vi "servo.vi"() -> ()   [LabVIEW 2023]
uses:
  <vilib>/Platform/TimedLoop/XDataNode/timing_clust.ctl
  <vilib>/Platform/TimedLoop/XDataNode/nitl_modes.ctl
  <vilib>/Platform/TimedLoop/XDataNode/wakeup.ctl
  <vilib>/Instr/_visa.llb/VISA Configure Serial Port (Instr).vi
  <vilib>/Utility/file.llb/Write Delimited Spreadsheet (DBL).vi
  <vilib>/Utility/file.llb/Write Delimited Spreadsheet (string).vi
  C:/Users/Ali/Desktop/ServoMotor/utilitytools39.dll
  utilitytools39.dll
  <vilib>/platform/TimedLoop/XDataNode/XDataNode.xnode
  <vilib>/Platform/TimedLoop/XDataNode/XDNodeRunTimeDep.lvlib
panel:
  out "Part":string
  out "ServoType":string
  in  "Speed Test":enum32{"A", "B"}(radio)
  out "final":string[][](array[string])
  out "k":dbl[](array[numeric])
  out "resultOfStep":dbl[](array[numeric])
  out "results":dbl[][](array[numeric])
  in  "Export And Save Data":bool
  in  "Title:":string
  out "Type":string[](array[string])
  out "stop var":bool
  out "Command":string
  out "SelectedType":bool
  out "SelectedPort":bool
  in  "Servo Motor PartNumber":string
  in  "Servo Motor type":string(combo)
  out "String 2":string
  in  "Select  Port":refnum<visa-resource-name>
  out "On/Off":bool
  in  "stop":bool
  in  "start":bool
  in  "Angle (degree)":i32(knob)=9 min=9 max=21 step=1 scale=9.0..21.0
  in  "Torque (N.m)":i32(slide) min=0 max=12 step=1 scale=0.0..12.0
  in  "Select":T1(radio)=enum."Torque Test"
  out "Angle":dbl(knob) scale=180.0..-180.0 scale format="%#_6f"
  out "Current (mA)":dbl(knob) scale=0.0..5500.0 scale format="%#_6f"
  out "Speed (degree/s)":dbl(knob) scale=0.0..600.0 scale format="%#_6f"
  out "Voltage  (volt)":dbl(knob) scale=0.0..25.0 scale format="%#_6f"
  out "Torque (N.M)":dbl(knob) scale=0.0..40.0 scale format="%#3.2f"
  # "Pishgaman Sanat Tissan  - Servo Motor Tester"
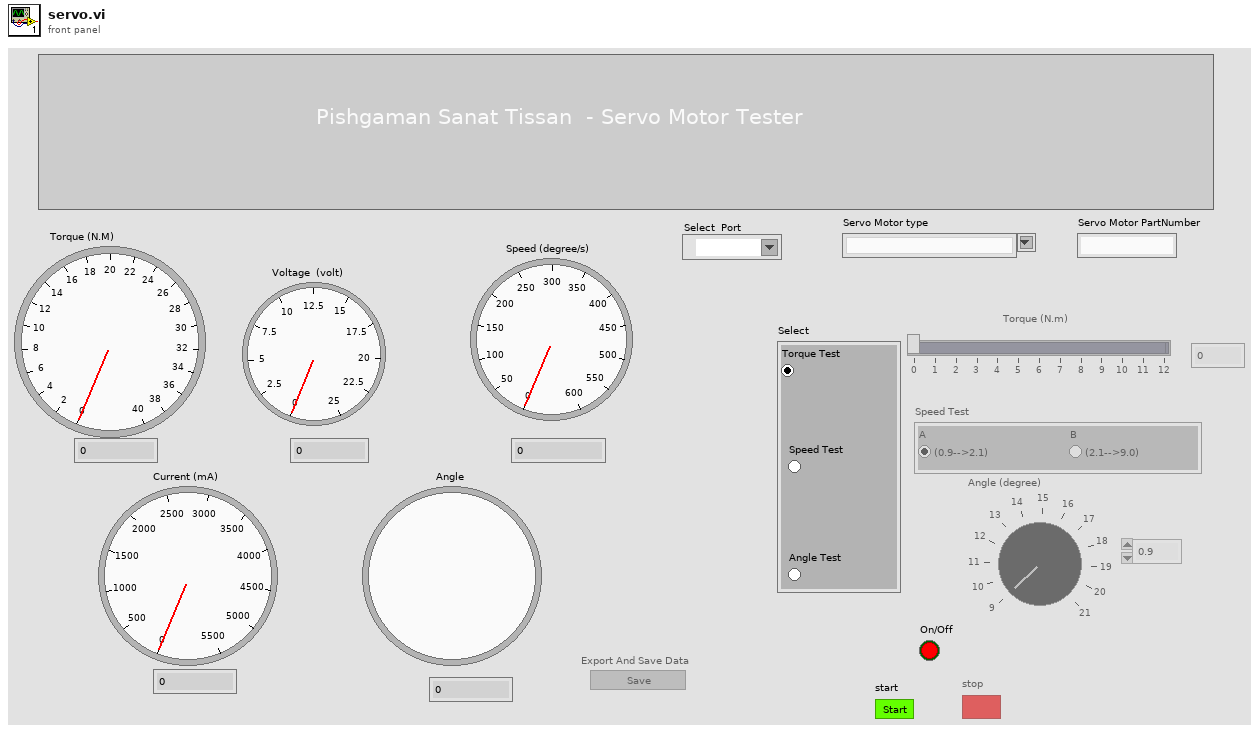
[diagram p1: front panel]
types:
  T1 = enum32{"No Selection", "Torque Test", "Speed Test", "Angle Test"}
  T2 = typedef "XDNodeRunTimeDep.lvlib/timing_clust.ctl" = cluster{"Expected End [f-1]":u64, "Actual End [f-1]":u64, "Finished Late? [f-1]":bool, "Expected End [i-1]":u64, "Actual End [i-1]":u64, "Finished Late? [i-1]":bool, "Expected Start [i]":u64, "Actual Start [i]":u64, "Expected Start [f]":u64, "Actual Start [f]":u64, "Source Name":string, "Structure Name":string, "Period":i64, "Deadline":i64, "Offset":i64, "Start":i64, "Priority":i32, "Timeout":i32, "Mode":T3, "Wakeup Reason":T4, "Error":errorcluster, "Source Type":string, "Secondary Source Type":string, "Global End Time":u64, "Global Start Time":u64, "Frame Duration":u64, "Iteration Duration":u64, "Assigned CPU":i32, "I/O Scan Engine Mode":u32}
  T3 = typedef "XDNodeRunTimeDep.lvlib/nitl_modes.ctl" = enum32{"No Change", "Process missed periods, maintain original phase", "Discard missed periods, maintain original phase", "Process missed periods, ignore original phase", "Discard missed periods, ignore original phase"}
  T4 = typedef "XDNodeRunTimeDep.lvlib/wakeup.ctl" = enum32{"Normal", "Aborted", "Asynchronous wakeup", "Timing source error", "Timed loop error", "Timeout"}
  T5 = typedef "LVDataSocketStatusTypeDef.ctl" = cluster{"Code":enum32{"Invalid Status", "Unconnected", "Active", "Idle", "Error", "Connecting"}, "Text":string}
  T6 = enum32{"Invalid Status", "Unconnected", "Active", "Idle", "Error", "Connecting"}
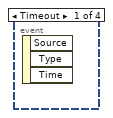
[diagram p2: hidden frame]
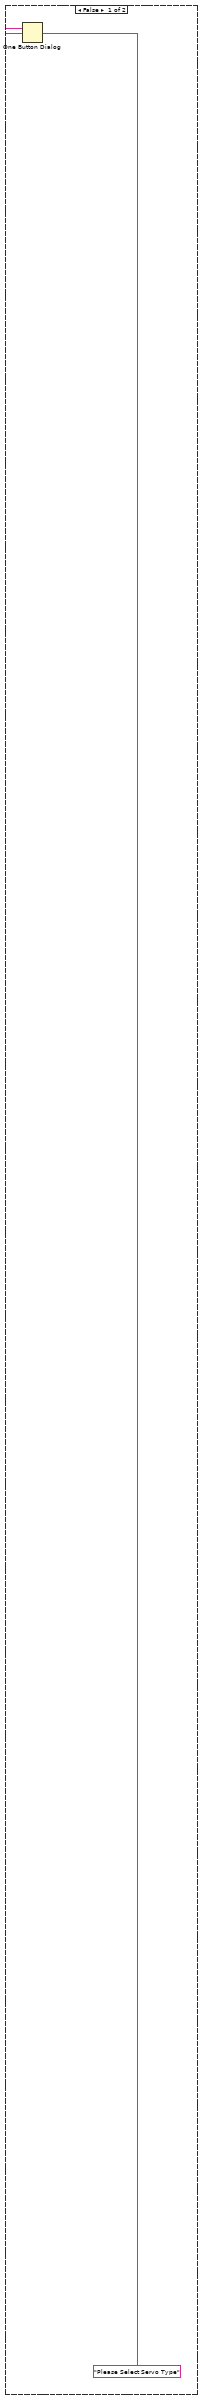
[diagram p4: hidden frame]
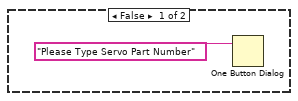
[diagram p5: hidden frame]
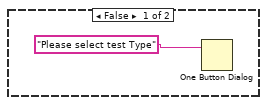
[diagram p6: hidden frame]
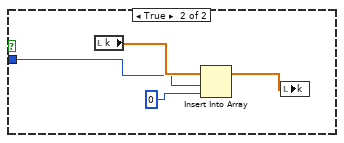
[diagram p7: hidden frame]
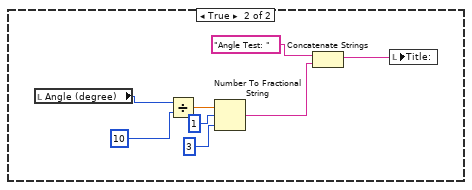
[diagram p12: hidden frame]
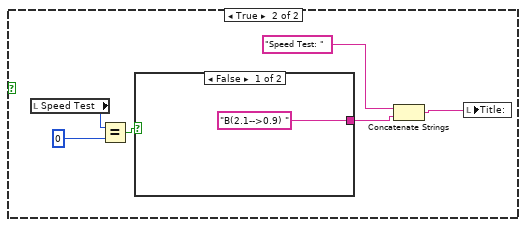
[diagram p13: hidden frame]
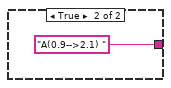
[diagram p14: hidden frame]
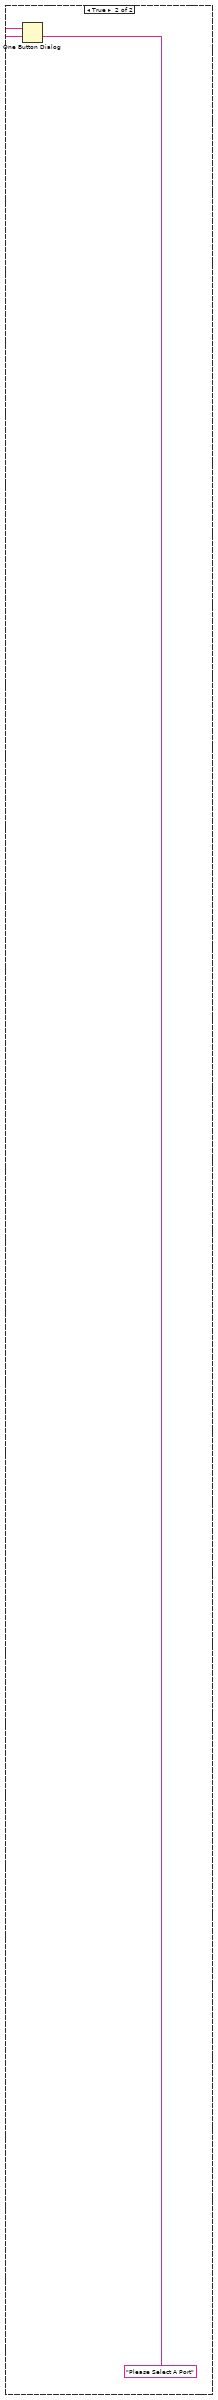
[diagram p17: hidden frame]
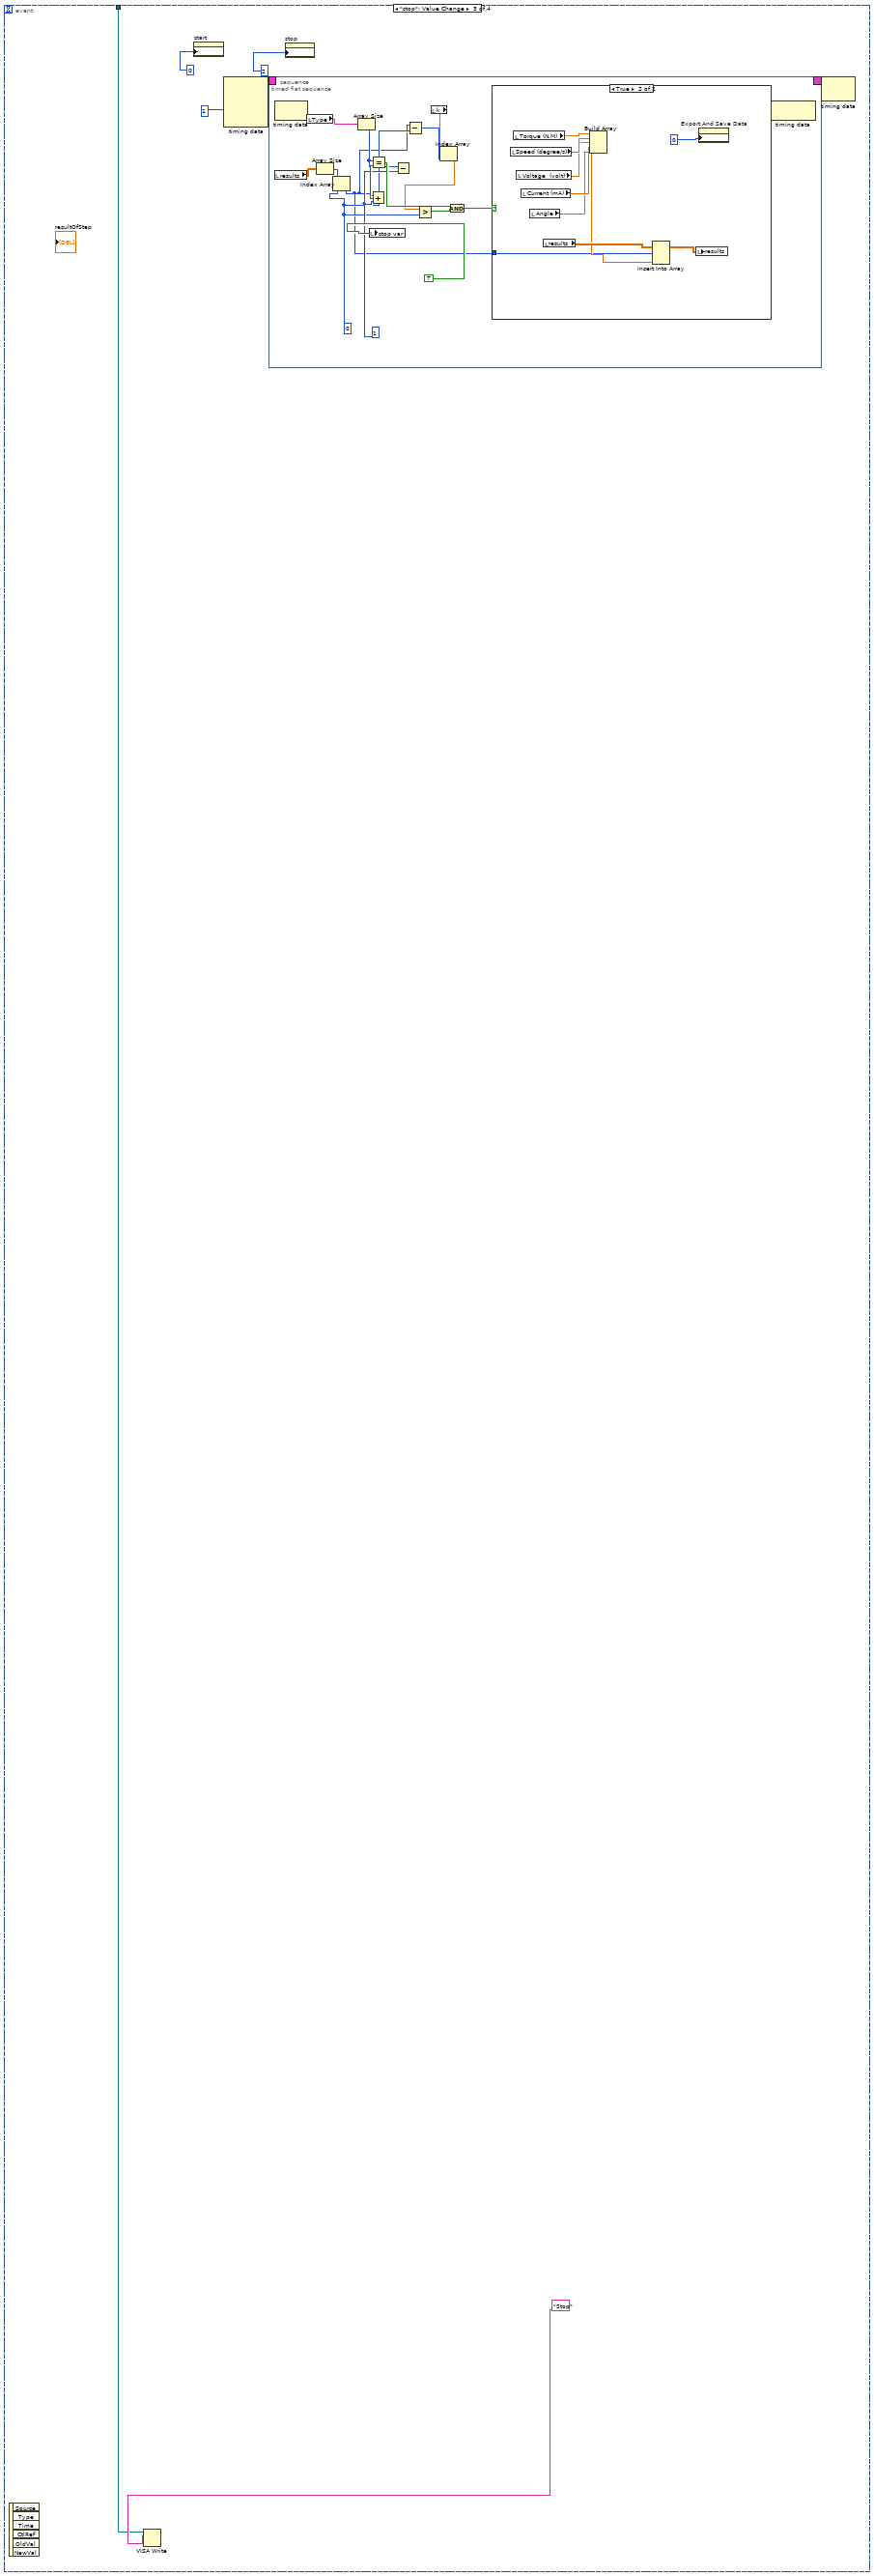
[diagram p18: hidden frame]
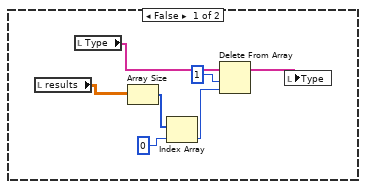
[diagram p19: hidden frame]
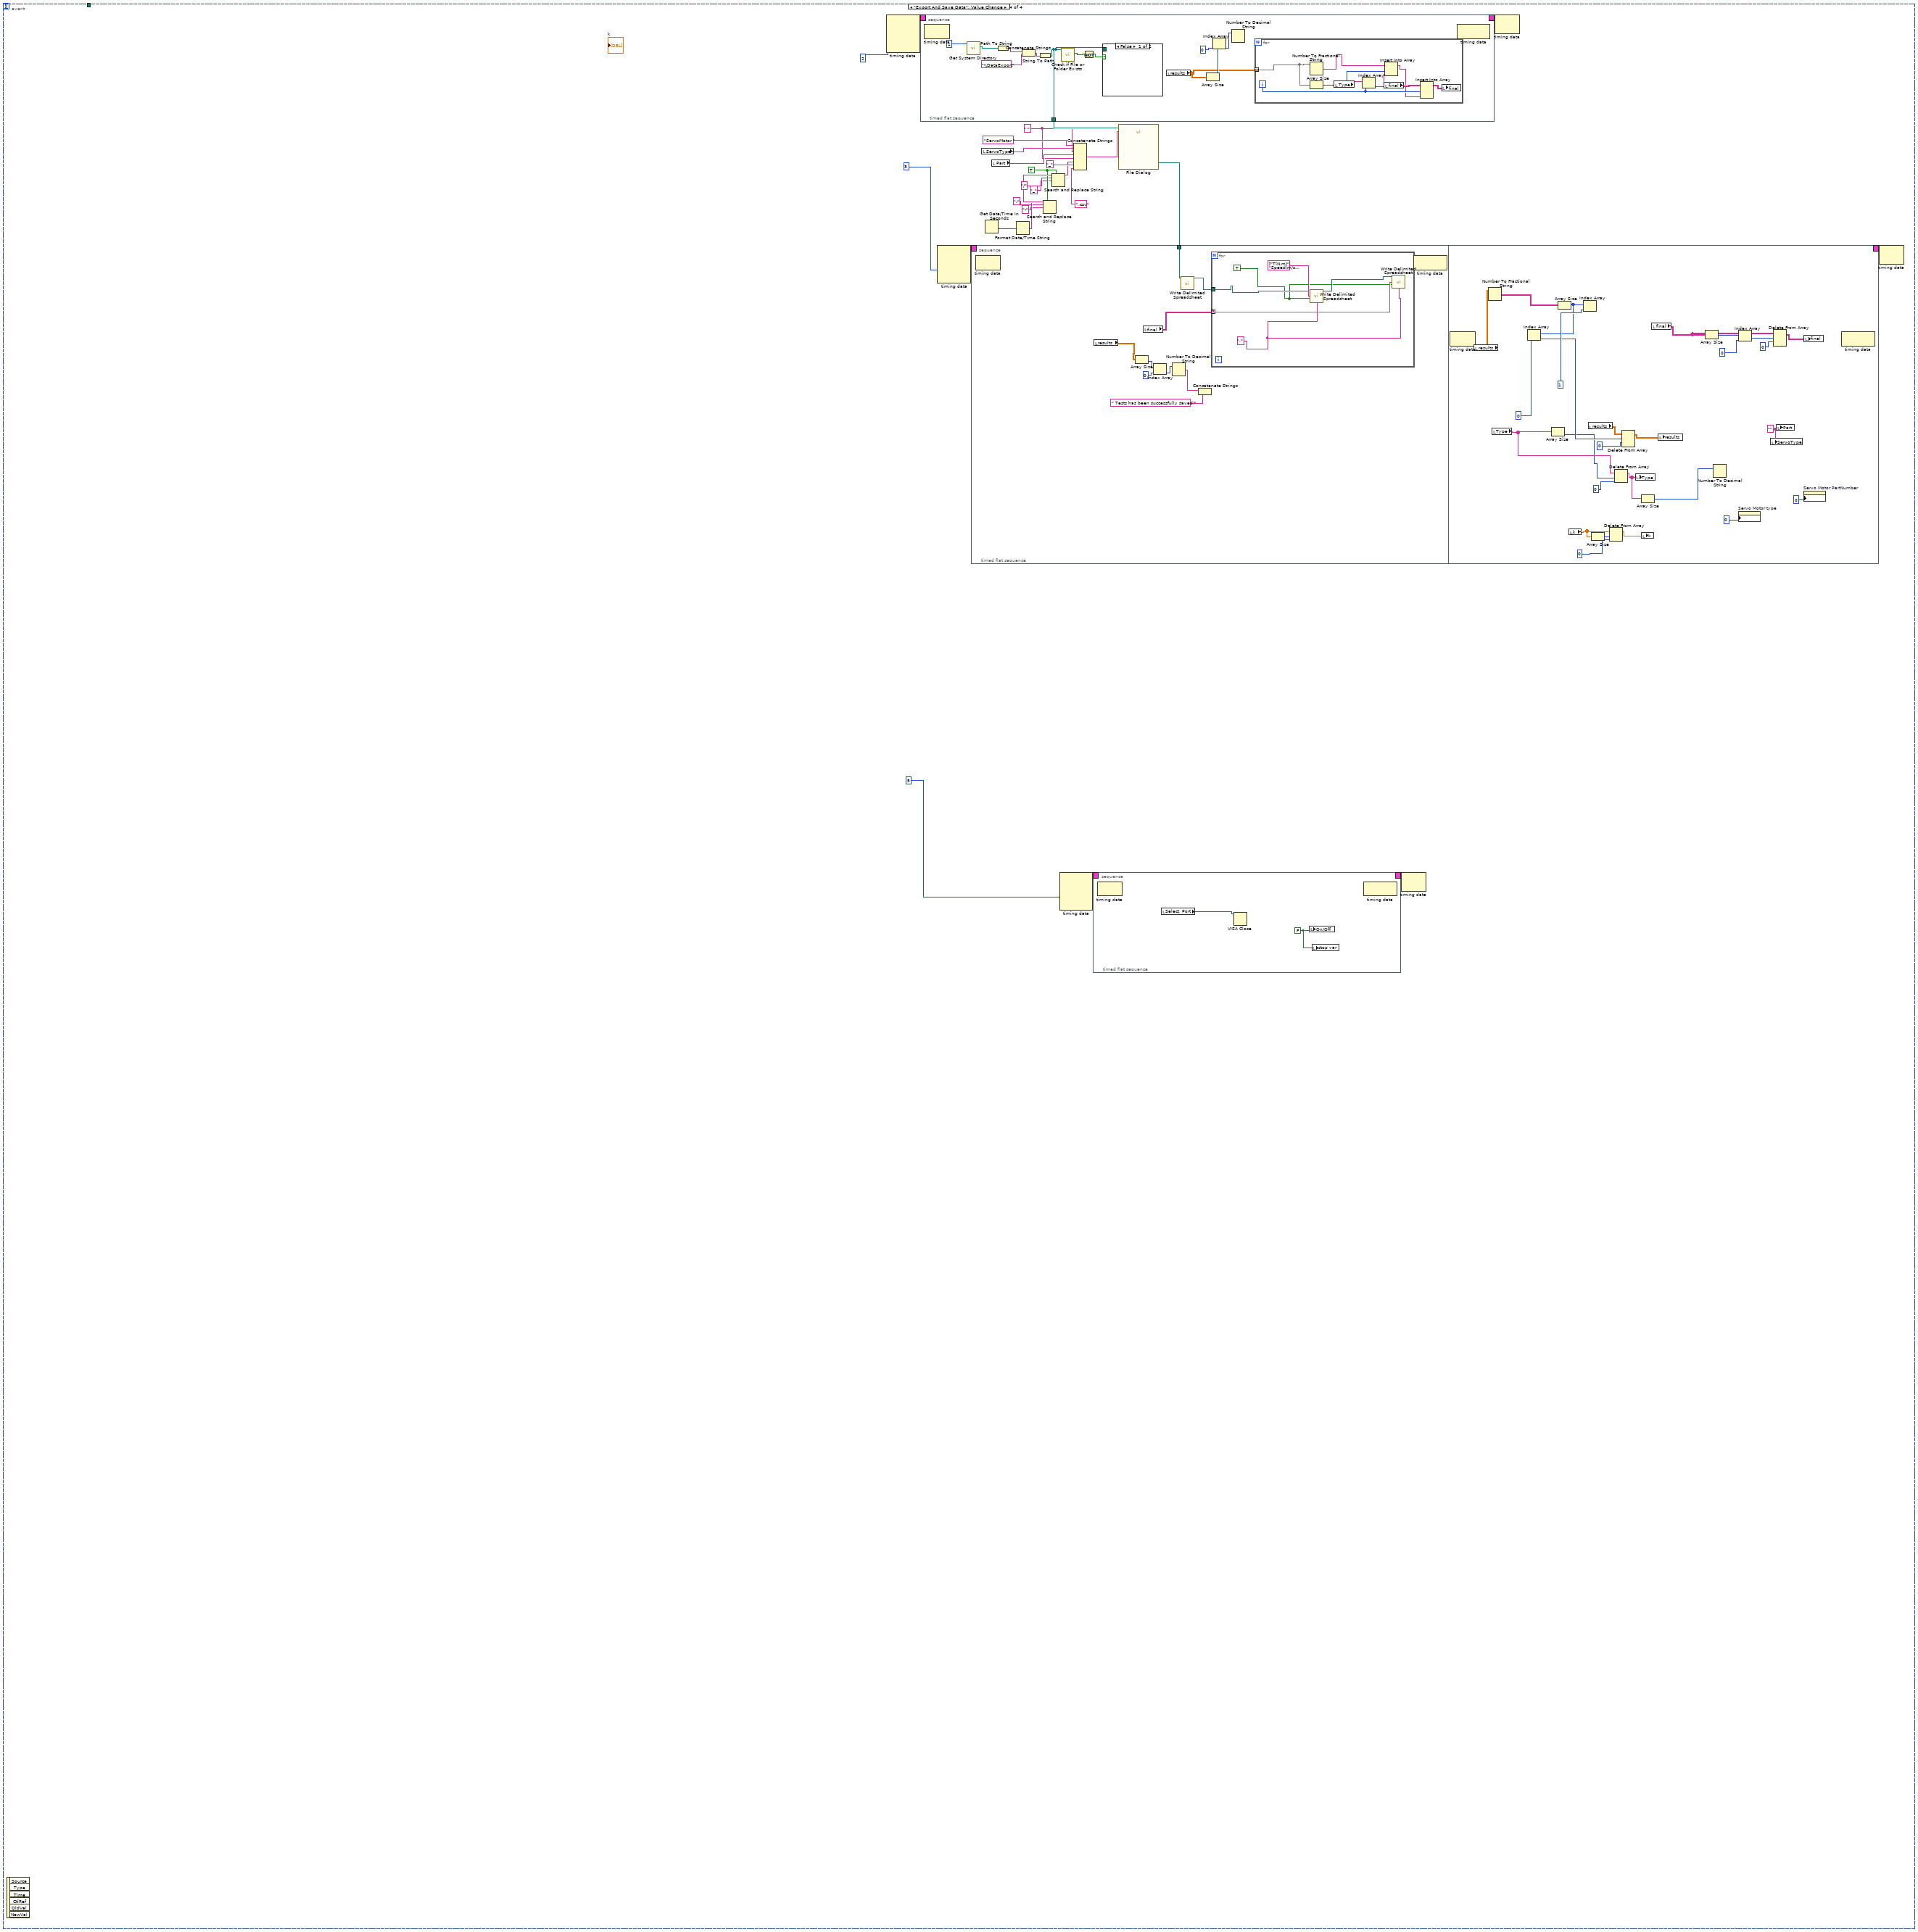
[diagram p20: hidden frame]
diagram:
  w1 = 0
  w10 = ""
  n1 = while {
    tunnel: "Select  Port" -> [w15]
    stop <- FALSE stop-if-true
    n2 = event shown="[1] \"start\": Value Change" {
      selector: _ -> [_ _ _ _]
      dyn-events: _ -> [_ _ _ _]
      timeout: _ -> [_ _ _ _]
      tunnel: w15 -> [_ w22 w155 _]
      tunnel: [_ w22 _ _] -> _
      event Timeout {
        n3 = event-data() -> ()  [unwired: 1 in, 3 out]
      }
      event "start": Value Change {
        w23 = ""
        n4 = event-data() -> ()  [unwired: 1 in, 6 out]
        n5 = local read "Select  Port"() -> (w25:refnum<visa-resource-name>)
        n6 = Concatenate Strings(w25, w23) -> (w24:string)
        n7 = property on="Select  Port" class="VISAName"() -> ("DtSktStatus"=w19:T5)  [unwired: 2 in, 2 out]
        n8 = Equal?(x=w24, y=w23) -> (x = y?=w20:bool)
        n9 = Not(x=w20) -> (.not. x?=w21:bool)
        n10 = local write "SelectedPort"(w21) -> ()
        n11 = case shown="False" w20 {
          tunnel: w22 -> [w29 _]
          frame False {
            n12 = local read "ServoType"() -> (w27:string)
            n13 = local read "Servo Motor type"() -> (w28:string)
            n14 = Not Equal?(x=w27, y="") -> (x != y?=w30:bool)
            n15 = local write "SelectedType"(w30) -> ()
            n16 = case shown="True" w30 {
              tunnel: w29 -> [_ w37]
              frame False {
                n17 = One Button Dialog(message="Please Select Servo Type") -> ()  [unwired: 1 in, 1 out]
              }
              frame True {
                n18 = local read "Servo Motor PartNumber"() -> (w34:string)
                n19 = local read "Part"() -> (w33:string)
                n20 = local write "Part"(w34) -> ()
                n21 = Not Equal?(x=w33, y="") -> (x != y?=w35:bool)
                n22 = case shown="True" w35 {
                  tunnel: w37 -> [_ w42]
                  frame False {
                    n23 = One Button Dialog(message="Please Type Servo Part Number") -> ()  [unwired: 1 in, 1 out]
                  }
                  frame True {
                    n24 = local read "Select"() -> (w39:T1)
                    n25 = Not Equal?(x=w39, y=0) -> (x != y?=w41:bool)
                    n26 = case shown="True" w41 {
                      tunnel: w42 -> [_ w66]
                      frame False {
                        n27 = One Button Dialog(message="Please select test Type") -> ()  [unwired: 1 in, 1 out]
                      }
                      frame True {
                        n28 = local read "results"() -> (w60:dbl[][])
                        n29 = local read "Type"() -> (w61:string[])
                        n30 = Array Size(array=w60) -> (size(s)=w59:i32[])
                        n31 = Index Array(array=w59, index=0) -> (element=w48:i32)
                        n32 = property on="Servo Motor PartNumber" class="Str"("DisabledEnum"=2) -> ()  [unwired: 2 in, 2 out]
                        n33 = Array Size(array=w61) -> (size(s)=w49:i32)
                        n34 = property on="Export And Save Data" class="Bool"("DisabledEnum"=2) -> ()  [unwired: 2 in, 2 out]
                        n35 = Add(x=w48, y=1) -> (x+y=w56:i32)
                        n36 = Equal?(x=w49, y=w56) -> (x = y?=w55:bool)
                        n37 = property on="start" class="Bool"("DisabledEnum"=2) -> ()  [unwired: 2 in, 2 out]
                        n38 = local read "Select"() -> (w68:T1)
                        n39 = property on="stop" class="Bool"("DisabledEnum"=0) -> ()  [unwired: 2 in, 2 out]
                        n40 = local read "stop var"() -> (w44:bool)
                        n41 = Equal?(x=w68, y=1) -> (x = y?=w52:bool)
                        n42 = case shown="True" w52 {
                          frame False {
                          }
                          frame True {
                            n43 = local read "Torque (N.m)"() -> (w144:i32)
                            n44 = Number To Decimal String(number=w144) -> (decimal integer string=w143:string)  [unwired: 1 in]
                            n45 = Concatenate Strings("Torque Test with: ", w143, " (N.m)") -> (w141:string)
                            n46 = local write "Title:"(w141) -> ()
                          }
                        }
                        n47 = case shown="False" w55 {
                          tunnel: w48 -> [_ w78]
                          frame False {
                            n48 = local read "results"() -> (w75:dbl[][])
                            n49 = local read "Type"() -> (w77:string[])
                            n50 = Array Size(array=w75) -> (size(s)=w74:i32[])
                            n51 = Index Array(array=w74, index=0) -> (element=w73:i32)
                            n52 = Delete From Array(array=w77, length=1, index=w73) -> (array with subset deleted=w76:string[])  [unwired: 1 out]
                            n53 = local write "Type"(w76) -> ()
                          }
                          frame True {
                            n54 = local read "k"() -> (w80:dbl[])
                            n55 = Insert Into Array(array=w80, index=w78, new element=0) -> (w81:dbl[])
                            n56 = local write "k"(w81) -> ()
                          }
                        }
                        n57 = case shown="False" w44 {
                          tunnel: w66 -> [w147 _]
                          frame False {
                            n58 = call-poly "VISA Configure Serial Port"("VISA resource name"=w147) -> ("VISA resource name out"=w146:refnum<visa-resource-name>)  [unwired: 13 in, 1 out]
                            n59 = VISA Write(VISA resource name=w146, write buffer="PST89") -> ()  [unwired: 1 in, 3 out]
                            n60 = VISA Open(VISA resource name=w146) -> ()  [unwired: 4 in, 2 out]
                          }
                          frame True {
                          }
                        }
                        n61 = local read "Type"() -> (w62:string[])
                        n62 = local read "Title:"() -> (w65:string)
                        n63 = property on="Servo Motor type" class="CmbBox"("DisabledEnum"=2) -> ()  [unwired: 2 in, 2 out]
                        n64 = Array Size(array=w62) -> (size(s)=w63:i32)
                        n65 = case shown="True" w44 {
                          tunnel: w66 -> [_ w83]
                          frame False {
                          }
                          frame True {
                            n66 = local read "Select"() -> (w84:T1)
                            n67 = Equal?(x=w84, y=3) -> (x = y?=w87:bool)
                            n68 = Equal?(x=w84, y=2) -> (x = y?=w86:bool)
                            n69 = Equal?(x=w84, y=1) -> (x = y?=w89:bool)
                            n70 = case shown="True" w89 {
                              frame False {
                              }
                              frame True {
                                n71 = local read "Torque (N.m)"() -> (w122:i32)
                                n72 = local read "ServoType"() -> (w114:string)
                                n73 = Divide(x=w122, y=10) -> (x/y=w121:dbl)
                                n74 = Number To Fractional String(number=w121, width (-)=3, precision (6)=1) -> (F-format string=w118:string)  [unwired: 1 in]
                                n75 = Concatenate Strings("@3", ",2,", w118, ",", w114, "#") -> (w123:string)
                                n76 = local write "Command"(w123) -> ()
                              }
                            }
                            n77 = case shown="True" w87 {
                              frame False {
                              }
                              frame True {
                                n78 = local read "Angle (degree)"() -> (w112:i32)
                                n79 = Divide(x=w112, y=10) -> (x/y=w107:dbl)
                                n80 = local read "ServoType"() -> (w103:string)
                                n81 = Number To Fractional String(number=w107, width (-)=3, precision (6)=1) -> (F-format string=w106:string)  [unwired: 1 in]
                                n82 = Concatenate Strings("@1", ",2,", w106, ",", w103, "#") -> (w109:string)
                                n83 = local write "Command"(w109) -> ()
                              }
                            }
                            n84 = case shown="True" w86 {
                              frame False {
                              }
                              frame True {
                                w92 = 0
                                w96 = ","
                                n85 = local read "Speed Test"() -> (w93:enum32{"A", "B"})
                                n86 = Subtract(x=w93, y=w92) -> (x-y=w91:u32)
                                n87 = Number To Decimal String(number=w91, width (-)=w92) -> (decimal integer string=w98:string)
                                n88 = local read "ServoType"() -> (w95:string)
                                n89 = Concatenate Strings("@2", w96, w98, w96, "0.0", w96, w95, "#") -> (w100:string)
                                n90 = local write "Command"(w100) -> ()
                              }
                            }
                            n91 = local read "Command"() -> (w82:string)
                            n92 = VISA Write(VISA resource name=w83, write buffer=w82) -> ()  [unwired: 1 in, 3 out]
                          }
                        }
                        n93 = Insert Into Array(array=w62, index=w63, new element=w65) -> (w64:string[])
                        n94 = Equal?(x=w68, y=2) -> (x = y?=w54:bool)
                        n95 = local write "Type"(w64) -> ()
                        n96 = case shown="False" w54 {
                          frame False {
                          }
                          frame True {
                            n97 = local read "Speed Test"() -> (w136:enum32{"A", "B"})
                            n98 = Equal?(x=w136, y=0) -> (x = y?=w137:bool)
                            n99 = case shown="False" w137 {
                              tunnel: ["B(2.1-->0.9) " "A(0.9-->2.1) "] -> w134
                              frame False {
                              }
                              frame True {
                              }
                            }
                            n100 = Concatenate Strings("Speed Test: ", w134) -> (w133:string)
                            n101 = local write "Title:"(w133) -> ()
                          }
                        }
                        n102 = Equal?(x=w68, y=3) -> (x = y?=w53:bool)
                        n103 = case shown="False" w53 {
                          frame False {
                          }
                          frame True {
                            n104 = local read "Angle (degree)"() -> (w131:i32)
                            n105 = Divide(x=w131, y=10) -> (x/y=w129:dbl)
                            n106 = Number To Fractional String(number=w129, width (-)=1, precision (6)=3) -> (F-format string=w126:string)  [unwired: 1 in]
                            n107 = Concatenate Strings("Angle Test: ", w126) -> (w125:string)
                            n108 = local write "Title:"(w125) -> ()
                          }
                        }
                      }
                    }
                  }
                }
              }
            }
            n109 = local write "ServoType"(w28) -> ()
          }
          frame True {
            n110 = One Button Dialog(message="Please Select A Port") -> ()  [unwired: 1 in, 1 out]
          }
        }
        n111 = Unbundle By Name(w19) -> ("Code"=w18:T6)
        n112 = Equal?(x=w18, y=0) -> (x = y?=w16:bool)
        n113 = case shown="True" w16 {
          frame False {
          }
          frame True {
            n114 = local write "On/Off"(TRUE) -> ()
          }
        }
      }
      event "stop": Value Change {
        n115 = event-data() -> ()  [unwired: 1 in, 6 out]
        n116 = VISA Write(VISA resource name=w155, write buffer="Stop") -> ()  [unwired: 1 in, 3 out]
        n117 = property on="start" class="Bool"("DisabledEnum"=0) -> ()  [unwired: 2 in, 2 out]
        n118 = node-c288(1) -> (w152:T2)  [unwired: 3 in]
        n119 = timed-sequence {
          timing: w152 -> [_]
          timing-out: [_] -> w151
          n120 = timed-flat-sequence {
            w160 = 1
            w158 = 0
            n121 = node-c288() -> ()  [unwired: 1 in, 1 out]
            n122 = local read "results"() -> (w170:dbl[][])
            n123 = local read "Type"() -> (w171:string[])
            n124 = Array Size(array=w170) -> (size(s)=w169:i32[])
            n125 = Index Array(array=w169, index=w158) -> (element=w157:i32)
            n126 = Array Size(array=w171) -> (size(s)=w162:i32)
            n127 = local write "stop var"(TRUE) -> ()
            n128 = Add(x=w157, y=w160) -> (x+y=w168:i32)
            n129 = Equal?(x=w162, y=w168) -> (x = y?=w166:bool)
            n130 = Subtract(x=w162, y=w160) -> ()  [unwired: 1 out]
            n131 = Subtract(x=w157, y=w158) -> (x-y=w159:i32)
            n132 = local read "k"() -> (w164:dbl[])
            n133 = Index Array(array=w164, index=w159) -> (element=w163:dbl)
            n134 = Greater?(x=w163, y=w158) -> (0:w167:bool)
            n135 = And(x=w166, y=w167) -> (x .and. y?=w165:bool)
            n136 = case shown="True" w165 {
              tunnel: w157 -> [_ w180]
              frame False {
                n137 = local read "results"() -> (w176:dbl[][])
                n138 = local read "Type"() -> (w178:string[])
                n139 = Array Size(array=w176) -> (size(s)=w175:i32[])
                n140 = Index Array(array=w175, index=0) -> (element=w173:i32)
                n141 = Delete From Array(array=w178, length=1, index=w173) -> (array with subset deleted=w177:string[])  [unwired: 1 out]
                n142 = local write "Type"(w177) -> ()
              }
              frame True {
                n143 = local read "Speed (degree/s)"() -> (w187:dbl)
                n144 = local read "Torque (N.M)"() -> (w188:dbl)
                n145 = local read "Voltage  (volt)"() -> (w186:dbl)
                n146 = local read "Current (mA)"() -> (w185:dbl)
                n147 = local read "Angle"() -> (w184:dbl)
                n148 = local read "results"() -> (w182:dbl[][])
                n149 = Build Array(w188, w187, w186, w185, w184) -> (w181:dbl[])
                n150 = Insert Into Array(array=w182, index (row)=w180, new element=w181) -> (w183:dbl[][])  [unwired: 1 in]
                n151 = local write "results"(w183) -> ()
                n152 = property on="Export And Save Data" class="Bool"("DisabledEnum"=0) -> ()  [unwired: 2 in, 2 out]
              }
            }
            n153 = node-c288() -> ()  [unwired: 1 in, 1 out]
          }
        }
        n154 = property on="stop" class="Bool"("DisabledEnum"=2) -> ()  [unwired: 2 in, 2 out]
        n155 = node-c288(w151) -> ()  [unwired: 1 out]
      }
      event "Export And Save Data": Value Change {
        w197 = " "
        w208 = TRUE
        n156 = event-data() -> ()  [unwired: 1 in, 6 out]
        n157 = node-c288(2) -> (w216:T2)  [unwired: 3 in]
        n158 = timed-sequence {
          timing: w216 -> [_]
          timing-out: [_] -> w215
          tunnel: [w222] -> w212
          n159 = timed-flat-sequence {
            tunnel: [w227] -> w222
            n160 = node-c288() -> ()  [unwired: 1 in, 1 out]
            n161 = call <vilib>:"Get System Directory.vi"("system directory type"=1) -> ("system directory"=w233:path)  [unwired: 10 in]
            n162 = Path To String(path=w233) -> (string=w232:string)
            n163 = Concatenate Strings(w232, "\\DataExport") -> (w230:string)
            n164 = String To Path(string=w230) -> (path=w227:path)
            n165 = call <vilib>:"Check if File or Folder Exists.vi"("path"=w227) -> ("file or folder exists?"=w229:bool)  [unwired: 8 in, 2 out]
            n166 = Not(x=w229) -> (.not. x?=w228:bool)
            n167 = case shown="False" w228 {
              tunnel: w227 -> [_ w244]
              frame False {
              }
              frame True {
                n168 = Create Folder(path (use dialog)=w244) -> ()  [unwired: 2 in, 3 out]
              }
            }
            n169 = local read "results"() -> (w224:dbl[][])
            n170 = Array Size(array=w224) -> (size(s)=w226:i32[])
            n171 = Index Array(array=w226, index=0) -> (element=w223:i32)
            n172 = Number To Decimal String(number=w223) -> ()  [unwired: 1 in, 1 out]
            n173 = for {
              tunnel: w224 -> [w235] mode=indexing
              i -> [w237]
              n174 = Array Size(array=w235) -> (size(s)=w242:i32)
              n175 = Number To Fractional String(number=w235) -> (F-format string=w243:string[])  [unwired: 3 in]
              n176 = local read "Type"() -> (w241:string[])
              n177 = Index Array(array=w241, index=w237) -> (element=w240:string)
              n178 = local read "final"() -> (w239:string[][])
              n179 = Insert Into Array "Insert Into Array"(array=w243, index=w242, new element=w240) -> (w236:string[])
              n180 = Insert Into Array(array=w239, index (row)=w237, new element=w236) -> (w238:string[][])  [unwired: 1 in]
              n181 = local write "final"(w238) -> ()
            }
            n182 = node-c288() -> ()  [unwired: 1 in, 1 out]
          }
        }
        n183 = node-c288(3) -> (w221:T2)  [unwired: 3 in]
        n184 = local read "ServoType"() -> (w200:string)
        n185 = Get Date/Time In Seconds() -> (seconds since 1Jan1904=w209:timestamp)
        n186 = local read "Part"() -> (w201:string)
        n187 = Format Date/Time String(seconds (now)=w209) -> (date/time string=w210:string)  [unwired: 2 in]
        n188 = Search and Replace String(replace all?=w208, input string=w210, search string=":", replace string="-") -> (result string=w211:string)  [unwired: 4 in, 3 out]
        n189 = Search and Replace String(replace all?=w208, input string=w211, search string="/", replace string="_") -> (result string=w204:string)  [unwired: 4 in, 3 out]
        n190 = node-c288(5) -> (w219:T2)  [unwired: 3 in]
        n191 = Concatenate Strings("ServoMotor ", w200, w197, w201, w197, w204, "_", ".csv") -> (w196:string)
        n192 = timed-sequence {
          timing: w219 -> [_]
          timing-out: [_] -> w218
          n193 = timed-flat-sequence {
            w251 = FALSE
            n194 = node-c288() -> ()  [unwired: 1 in, 1 out]
            n195 = local read "Select  Port"() -> (w252:refnum<visa-resource-name>)
            n196 = VISA Close(VISA resource name=w252) -> ()  [unwired: 1 in, 1 out]
            n197 = local write "On/Off"(w251) -> ()
            n198 = local write "stop var"(w251) -> ()
            n199 = node-c288() -> ()  [unwired: 1 in, 1 out]
          }
        }
        n200 = call "File Dialog"("start path"=w212, "default name"=w196) -> ("selected path"=w195:path)  [unwired: 10 in, 3 out]
        n201 = timed-sequence {
          timing: w221 -> [_]
          timing-out: [_] -> w220
          tunnel: w195 -> [w259]
          n202 = timed-flat-sequence {
            tunnel: w259 -> [w260]
            frame #0 {
              n203 = node-c288() -> ()  [unwired: 1 in, 1 out]
              n204 = local read "results"() -> (w263:dbl[][])
              n205 = Array Size(array=w263) -> (size(s)=w266:i32[])
              n206 = local read "final"() -> (w267:string[][])
              n207 = Index Array(array=w266, index=0) -> (element=w264:i32)
              n208 = Number To Decimal String(number=w264) -> (decimal integer string=w262:string)  [unwired: 1 in]
              n209 = call-poly <vilib>:"Write Delimited Spreadsheet.vi"("file path (dialog if empty)"=w260) -> ("new file path (Not A Path if cancelled)"=w268:path)  [unwired: 13 in, 1 out]
              n210 = Concatenate Strings(w262, " Tests has been successfully saved!") -> ()  [unwired: 1 out]
              n211 = for {
                tunnel: w268 -> [w273]
                tunnel: w267 -> [w270] mode=indexing
                w271 = ","
                w269 = TRUE
                n212 = call-poly <vilib>:"Write Delimited Spreadsheet.vi"("file path (dialog if empty)"=w273, "1D data"=string[] ["T(N.m)", "Speed(m/s)", "Voltage (volt)", "Current (mA)", "Angle (degree)"], "append to file? (new file:F)"=w269, "delimiter (\\t)"=w271) -> ("new file path (Not A Path if cancelled)"=w272:path)  [unwired: 10 in, 1 out]
                n213 = call-poly <vilib>:"Write Delimited Spreadsheet.vi"("file path (dialog if empty)"=w272, "1D data"=w270, "append to file? (new file:F)"=w269, "delimiter (\\t)"=w271) -> ()  [unwired: 10 in, 2 out]
              }
              n214 = node-c288() -> ()  [unwired: 1 in, 1 out]
            }
            frame #1 {
              w277 = ""
              n215 = node-c288() -> ()  [unwired: 1 in, 1 out]
              n216 = local read "results"() -> (w289:dbl[][])
              n217 = Number To Fractional String(number=w289) -> (F-format string=w288:string[][])  [unwired: 3 in]
              n218 = local read "Type"() -> (w292:string[])
              n219 = Array Size(array=w292) -> (size(s)=w296:i32)
              n220 = Array Size(array=w288) -> (size(s)=w302:i32[])
              n221 = Index Array "Index Array"(array=w302, index=0) -> (element=w299:i32)
              n222 = local read "k"() -> (w294:dbl[])
              n223 = Index Array(array=w302, index=1) -> ()  [unwired: 1 out]
              n224 = local read "results"() -> (w300:dbl[][])
              n225 = Array Size(array=w294) -> (size(s)=w295:i32)
              n226 = Delete From Array(array=w294, length=w295, index=0) -> (array with subset deleted=w280:dbl[])  [unwired: 1 out]
              n227 = Delete From Array(array=w292, length=w296, index=0) -> (array with subset deleted=w291:string[])  [unwired: 1 out]
              n228 = Delete From Array "Delete From Array"(array=w300, length=w299, index (row)=0) -> (array with subset deleted=w281:dbl[][])  [unwired: 1 in, 1 out]
              n229 = local write "Type"(w291) -> ()
              n230 = Array Size(array=w291) -> (size(s)=w290:i32)
              n231 = local write "k"(w280) -> ()
              n232 = local read "final"() -> (w285:string[][])
              n233 = local write "results"(w281) -> ()
              n234 = Array Size(array=w285) -> (size(s)=w287:i32[])
              n235 = Number To Decimal String(number=w290) -> ()  [unwired: 1 in, 1 out]
              n236 = Index Array(array=w287, index=0) -> (element=w284:i32)
              n237 = property on="Servo Motor type" class="CmbBox"("DisabledEnum"=0) -> ()  [unwired: 2 in, 2 out]
              n238 = local write "ServoType"(w277) -> ()
              n239 = Delete From Array(array=w285, length=w284, index (row)=0) -> (array with subset deleted=w282:string[][])  [unwired: 1 in, 1 out]
              n240 = local write "Part"(w277) -> ()
              n241 = property on="Servo Motor PartNumber" class="Str"("DisabledEnum"=0) -> ()  [unwired: 2 in, 2 out]
              n242 = local write "final"(w282) -> ()
              n243 = node-c288() -> ()  [unwired: 1 in, 1 out]
            }
          }
        }
        n244 = node-c288(w218) -> ()  [unwired: 1 out]
        n245 = node-c288(w215) -> ()  [unwired: 1 out]
        n246 = node-c288(w220) -> ()  [unwired: 1 out]
      }
    }
  }
  n247 = while {
    stop <- FALSE stop-if-true
    n248 = Equal?(x="Select", y=1) -> (x = y?=w315:bool)
    n249 = Equal?(x="Select", y=2) -> (x = y?=w317:bool)
    n250 = case shown="True" w315 {
      frame False {
        n251 = property on="Torque (N.m)" class="Slide (strict)"("DisabledEnum"=2) -> ()  [unwired: 2 in, 2 out]
      }
      frame True {
        n252 = property on="Torque (N.m)" class="Slide (strict)"("DisabledEnum"=0) -> ()  [unwired: 2 in, 2 out]
      }
    }
    n253 = case shown="False" w317 {
      frame False {
        n254 = property on="Speed Test" class="RadioBtnsControl (strict)"("DisabledEnum"=2) -> ()  [unwired: 2 in, 2 out]
      }
      frame True {
        n255 = property on="Speed Test" class="RadioBtnsControl (strict)"("DisabledEnum"=0) -> ()  [unwired: 2 in, 2 out]
      }
    }
    n256 = Equal?(x="Select", y=3) -> (x = y?=w311:bool)
    n257 = case shown="False" w311 {
      frame False {
        n258 = property on="Angle (degree)" class="Knob (strict)"("DisabledEnum"=2) -> ()  [unwired: 2 in, 2 out]
      }
      frame True {
        n259 = property on="Angle (degree)" class="Knob (strict)"("DisabledEnum"=0) -> ()  [unwired: 2 in, 2 out]
      }
    }
  }
  n260 = local read "Select  Port"() -> (w12:refnum<visa-resource-name>)
  n261 = local write "stop var"(FALSE) -> ()
  n262 = property on="start" class="Bool"("DisabledEnum"=0) -> ()  [unwired: 2 in, 2 out]
  n263 = property on="stop" class="Bool"("DisabledEnum"=2) -> ()  [unwired: 2 in, 2 out]
  n264 = Concatenate Strings(w12, w10) -> (w11:string)
  n265 = Equal?(x=w11, y=w10) -> (x = y?=w8:bool)
  n266 = Not(x=w8) -> (.not. x?=→"SelectedPort":bool)
  n267 = case shown="False" w8 {
    frame False {
    }
    frame True {
      n268 = One Button Dialog(message="Please Select A Port") -> ()  [unwired: 1 in, 1 out]
    }
  }
  n269 = property on="Export And Save Data" class="Bool"("DisabledEnum"=2) -> ()  [unwired: 2 in, 2 out]
  n270 = property on="Servo Motor type" class="CmbBox"("DisabledEnum"=w1) -> ()  [unwired: 2 in, 2 out]
  n271 = property on="Servo Motor PartNumber" class="Str"("DisabledEnum"=w1) -> ()  [unwired: 2 in, 2 out]
  n272 = local read "SelectedPort"() -> (w7:bool)
  n273 = Not(x=w7) -> (.not. x?=w6:bool)
  n274 = while {
    tunnel: "Select  Port" -> [w326]
    tunnel: w6 -> [w328]
    stop <- w328 stop-if-true
    n275 = local read "SelectedPort"() -> (w327:bool)
    n276 = case shown="True" w327 {
      tunnel: w326 -> [_ w336]
      tunnel: [0 w335] -> w325
      frame False {
      }
      frame True {
        n277 = property class="Instr"(reference=w336) -> ("Serial Settings:Number of Bytes at Serial Port"=w335:u32)  [unwired: 1 in, 2 out]
      }
    }
    n278 = Wait (ms)(milliseconds to wait=1500) -> ()  [unwired: 1 out]
    n279 = Greater?(x=w325, y=0) -> (0:w332:bool)
    n280 = Add(x=w325, y=0) -> (x+y=w331:u32)
    n281 = case shown="True" w332 {
      tunnel: w326 -> [_ w341]
      tunnel: w325 -> [_ _]
      tunnel: w331 -> [_ w340]
      frame False {
      }
      frame True {
        n282 = VISA Read(VISA resource name=w341, byte count=w340) -> (read buffer=w338:string)  [unwired: 1 in, 3 out]
        "String 2" <- w338
        n283 = Equal?(x=w338, y="PassOk") -> (x = y?=w337:bool)
        n284 = case shown="False" w337 {
          tunnel: w341 -> [_ w374]
          tunnel: w338 -> [w345 _]
          tunnel: w337 -> [_ w372]
          frame False {
            n285 = constructor class="SerialPortCom"() -> (reference out=w346:refnum<k24>)  [unwired: 3 in, 2 out]
            n286 = String Length(string=w345) -> (length=w343:i32)
            n287 = Greater?(x=w343, y=19) -> (0:w344:bool)
            n288 = case shown="True" w344 {
              tunnel: w346 -> [_ w371]
              tunnel: w345 -> [_ w370]
              frame False {
              }
              frame True {
                n289 = local read "results"() -> (w356:dbl[][])
                n290 = local read "k"() -> (w351:dbl[])
                n291 = invoke class="SerialPortCom" method="Read"(reference=w371, "str"=w370) -> ("Read"=w360:dbl[])  [unwired: 2 in, 3 out]
                n292 = local read "k"() -> (w357:dbl[])
                n293 = Array Size(array=w356) -> (size(s)=w355:i32[])
                n294 = Index Array(array=w355, index=0) -> (element=w353:i32)
                n295 = Subtract(x=w353, y=0) -> (x-y=w350:i32)
                n296 = Index Array(array=w351, index=w350) -> (element=w349:dbl)
                n297 = Add(x=w349, y=1) -> (x+y=w347:dbl)
                n298 = Insert Into Array "Insert Into Array"(array=w357, index=w350, new element=w347) -> (w358:dbl[])
                n299 = local write "k"(w358) -> ()
                n300 = Index Array(array=w360, index=0) -> (element=→"Torque (N.M)":dbl)
                n301 = Index Array(array=w360, index=1) -> (element=→"Voltage  (volt)":dbl)
                n302 = Index Array(array=w360, index=3) -> (element=→"Angle":dbl)
                n303 = Index Array(array=w360, index=4) -> (element=→"Speed (degree/s)":dbl)
                n304 = Index Array(array=w360, index=2) -> (element=→"Current (mA)":dbl)
              }
            }
          }
          frame True {
            n305 = local write "On/Off"(TRUE) -> ()
            n306 = Concatenate Strings("You are susseccfuly connected to port:", w374) -> (w375:string)
            n307 = One Button Dialog(message=w375) -> ()  [unwired: 1 in, 1 out]
            n308 = case shown="True" w372 {
              tunnel: w374 -> [_ w385]
              frame False {
              }
              frame True {
                n309 = local read "Select"() -> (w378:T1)
                n310 = local read "Command"() -> (w377:string)
                n311 = Equal?(x=w378, y=3) -> (x = y?=w381:bool)
                n312 = Equal?(x=w378, y=2) -> (x = y?=w380:bool)
                n313 = Equal?(x=w378, y=1) -> (x = y?=w383:bool)
                n314 = case shown="True" w383 {
                  frame False {
                  }
                  frame True {
                    n315 = local read "Torque (N.m)"() -> (w417:i32)
                    n316 = local read "ServoType"() -> (w409:string)
                    n317 = Divide(x=w417, y=10) -> (x/y=w416:dbl)
                    n318 = Number To Fractional String(number=w416, width (-)=3, precision (6)=1) -> (F-format string=w413:string)  [unwired: 1 in]
                    n319 = Concatenate Strings("@3", ",2,", w413, ",", w409, "#") -> (w418:string)
                    n320 = local write "Command"(w418) -> ()
                  }
                }
                n321 = VISA Write(VISA resource name=w385, write buffer=w377) -> ()  [unwired: 1 in, 3 out]
                n322 = case shown="True" w381 {
                  frame False {
                  }
                  frame True {
                    n323 = local read "Angle (degree)"() -> (w407:i32)
                    n324 = Divide(x=w407, y=10) -> (x/y=w402:dbl)
                    n325 = local read "ServoType"() -> (w398:string)
                    n326 = Number To Fractional String(number=w402, width (-)=3, precision (6)=1) -> (F-format string=w401:string)  [unwired: 1 in]
                    n327 = Concatenate Strings("@1", ",2,", w401, ",", w398, "#") -> (w404:string)
                    n328 = local write "Command"(w404) -> ()
                  }
                }
                n329 = case shown="True" w380 {
                  frame False {
                  }
                  frame True {
                    w387 = 0
                    w391 = ","
                    n330 = local read "Speed Test"() -> (w388:enum32{"A", "B"})
                    n331 = Subtract(x=w388, y=w387) -> (x-y=w386:u32)
                    n332 = Number To Decimal String(number=w386, width (-)=w387) -> (decimal integer string=w393:string)
                    n333 = local read "ServoType"() -> (w390:string)
                    n334 = Concatenate Strings("@2", w391, w393, w391, "0.0", w391, w390, "#") -> (w395:string)
                    n335 = local write "Command"(w395) -> ()
                  }
                }
              }
            }
          }
        }
      }
    }
  }
